vi "Configure RF Output.vi"(4 "Enable Reverse Power Protection (T:Enable)":bool=TRUE, 6 "Enable Blanking (T:Enable)":bool=TRUE, 7 "Enable Modulation (T:Enable)":bool=TRUE, 8 "error in (no error)":errorcluster, 9 "Auto Blanking (T:Enable)":bool=TRUE, 10 "Enable RF Output (F:Disable)":bool, 11 "VISA resource name":refnum<visa-resource-name>) -> (0 "error out":errorcluster, 3 "VISA resource name out":refnum<visa-resource-name>)   [LabVIEW 2011, in "Agilent PSG MXG Series.lvlib"]
doc: "Configures RF output, modulation state, blanking, and RPP circuit of the signal generator."
uses:
  Agilent PSG MXG Series.lvlib
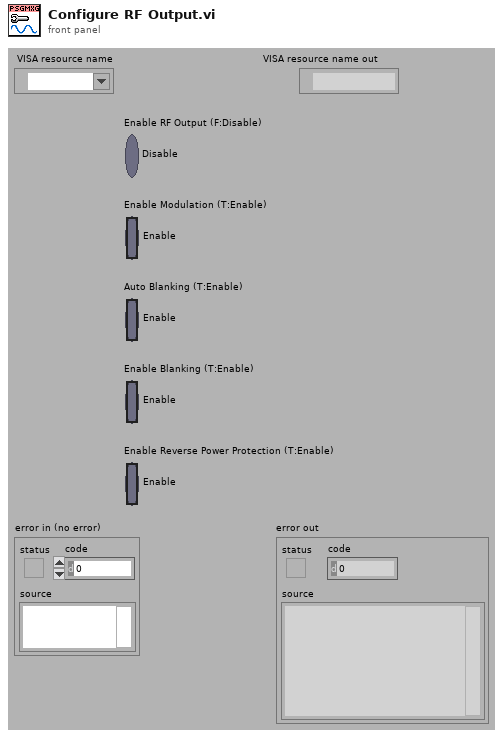
[diagram p1: front panel]
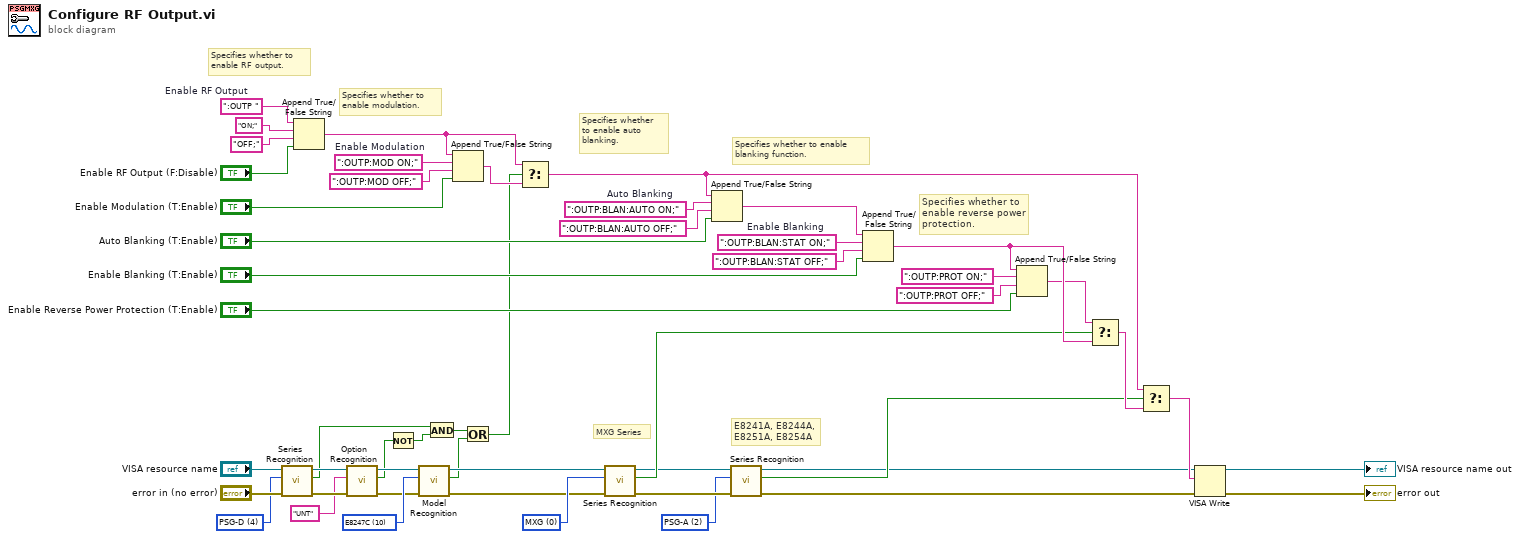
[diagram p0: block diagram]
diagram:
  w14 = u16 4 items=["MXG", "PSG", "PSG-A", "PSG-C", "PSG-D"] ("Series Type (0: MXG)")
  w22 = u16 10 items=["N5181A"=0, "N5182A"=1, "E8241A"=5, "E8244A"=6, "E8251A"=7, "E8254A"=8, "E8247C"=10, "E8257C"=11, "E8267C"=12, "E8257D"=15, "E8267D"=16] ("Model Type (0: N5181A)")
  w23 = u16 2 items=["MXG", "PSG", "PSG-A", "PSG-C", "PSG-D"] ("Series Type (0: MXG)")
  w24 = u16 0 items=["MXG", "PSG", "PSG-A", "PSG-C", "PSG-D"] ("Series Type (0: MXG)")
  w31 = ":OUTP:BLAN:STAT ON;"  # Enable Blanking
  w44 = ":OUTP:BLAN:AUTO ON;"  # Auto Blanking
  w47 = ":OUTP:MOD ON;"  # Enable Modulation
  w51 = ":OUTP "  # Enable RF Output
  # "MXG Series"
  # "Specifies whether to\nenable reverse power\nprotection."
  # "Specifies whether to enable\nblanking function."
  # "Specifies whether\nto enable auto\nblanking."
  # "Specifies whether to\nenable modulation."
  # "Specifies whether to\nenable RF output."
  # "E8241A, E8244A,\nE8251A, E8254A"
  n1 = call "Series Recognition.vi"("error in (no error)"="error in (no error)", "Series Type (0: MXG)"=w14, "VISA resource name"="VISA resource name") -> ("error out"=w12:errorcluster, "Is Series Correct"=w6:bool, "VISA resource name out"=w13:refnum<visa-resource-name>)  [unwired: 6 in]
  n2 = Append True/False String(1:"Enable RF Output (F:Disable)", 2:"OFF;" ("false string"), 3:"ON;" ("true string"), 4:w51) -> (0:w21:string)
  n3 = call "Option Recognition.vi"("error in (no error)"=w12, "Option (\"\")"="UNT" ("Option (\"\")"), "VISA resource name"=w13) -> ("error out"=w9:errorcluster, "Is Option Installed"=w8:bool, "VISA resource name out"=w10:refnum<visa-resource-name>)  [unwired: 6 in]
  n4 = Not(x=w8) -> (.not. x?=w7:bool)
  n5 = call "Model Recognition.vi"("error in (no error)"=w9, "Model Type (0: N5181A)"=w22, "VISA resource name"=w10) -> ("error out"=w17:errorcluster, "Is Model Correct"=w4:bool, "VISA resource name out"=w18:refnum<visa-resource-name>)  [unwired: 6 in]
  n6 = And(x=w6, y=w7) -> (x .and. y?=w5:bool)
  n7 = Append True/False String(1:"Enable Modulation (T:Enable)", 2:":OUTP:MOD OFF;" ("true string"), 3:w47, 4:w21) -> (0:w20:string)
  n8 = Or(x=w5, y=w4) -> (x .or. y?=w3:bool)
  n9 = Select(t=w21, s=w3, f=w20) -> (s? t:f=w19:string)
  n10 = call "Series Recognition.vi"("error in (no error)"=w17, "Series Type (0: MXG)"=w24, "VISA resource name"=w18) -> ("error out"=w28:errorcluster, "Is Series Correct"=w30:bool, "VISA resource name out"=w29:refnum<visa-resource-name>)  [unwired: 6 in]
  n11 = Append True/False String(1:"Auto Blanking (T:Enable)", 2:":OUTP:BLAN:AUTO OFF;" ("true string"), 3:w44, 4:w19) -> (0:w41:string)
  n12 = call "Series Recognition.vi"("error in (no error)"=w28, "Series Type (0: MXG)"=w23, "VISA resource name"=w29) -> ("error out"=w25:errorcluster, "Is Series Correct"=w27:bool, "VISA resource name out"=w26:refnum<visa-resource-name>)  [unwired: 6 in]
  n13 = Append True/False String(1:"Enable Blanking (T:Enable)", 2:":OUTP:BLAN:STAT OFF;" ("true string"), 3:w31, 4:w41) -> (0:w35:string)
  n14 = Append True/False String(1:"Enable Reverse Power Protection (T:Enable)", 2:":OUTP:PROT OFF;" ("true string"), 3:":OUTP:PROT ON;" ("Enable Reverse Power Protection"), 4:w35) -> (0:w34:string)
  n15 = Select(t=w34, s=w30, f=w35) -> (s? t:f=w33:string)
  n16 = Select(t=w19, s=w27, f=w33) -> (s? t:f=w32:string)
  n17 = VISA Write(VISA resource name=w26, write buffer=w32, error in (no error)=w25) -> (VISA resource name out=→"VISA resource name out":refnum<visa-resource-name>, error out=→"error out":errorcluster)  [unwired: 1 out]
